vi "账户保存.vi"(8 "error in (no error)":errorcluster caption="错误输入（无错误）", 10 "密码":string="018108ssl", 11 "账户名":string="SunSuoli") -> (0 "error out":errorcluster caption="错误输出")   [LabVIEW 2018]
uses:
  <vilib>/Utility/config.llb/Write Key (String).vi
  <vilib>/Utility/config.llb/NI_LVConfig.lvlib
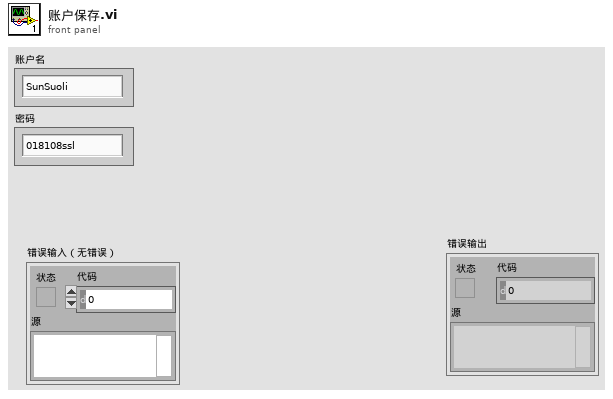
[diagram p1: front panel]
types:
  T1 = typedef "NI_LVConfig.lvlib/Config Data RefNum.ctl" = refnum<k1>
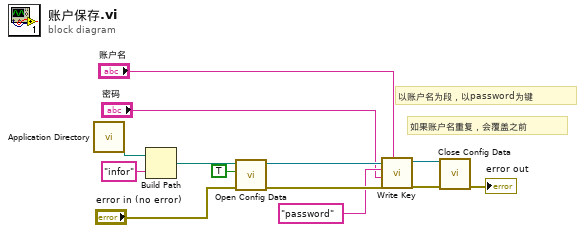
[diagram p0: block diagram]
diagram:
  # "如果账户名重复，会覆盖之前"
  # "以账户名为段，以password为键"
  n1 = call <vilib>:"Application Directory.vi"() -> ("Application Directory"=w12:path)
  n2 = Build Path(base path=w12, name or relative path="infor" ("名称或相对路径")) -> (appended path=w11:path)
  n3 = call <vilib>:"Open Config Data.vi"("error in (no error)"="error in (no error)", "create file if necessary (T)"=TRUE, "configuration file path"=w11) -> ("error out"=w8:errorcluster, "refnum"=w10:T1)  [unwired: 6 in, 1 out]
  n4 = call-poly <vilib>:"Write Key.vi"("section"="账户名", "error in (no error)"=w8, "value"="密码", "key"="password", "refnum"=w10) -> ("error out"=w4:errorcluster, "refnum out"=w5:T1)  [unwired: 4 in, 1 out]
  n5 = call <vilib>:"Close Config Data.vi"("error in (no error)"=w4, "refnum"=w5) -> ("error out"=→"error out":errorcluster)  [unwired: 8 in, 1 out]
